vi "Error.Compare Errors with No Error Opt if Same.vi"(7 "No Error if Same":bool=TRUE, 10 "error in2":errorcluster, 11 "error in1":errorcluster) -> (2 "error out":errorcluster, 3 "Same":bool)   [LabVIEW 2018]
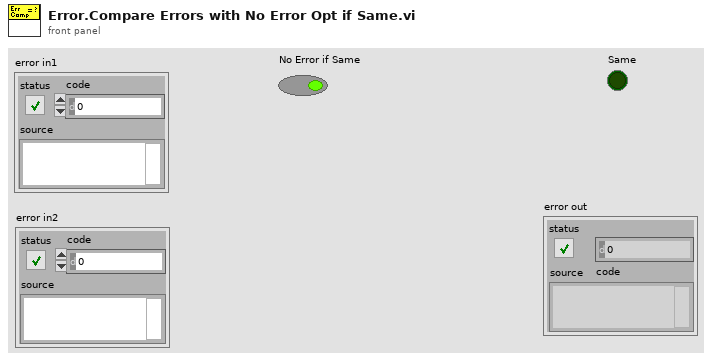
[diagram p1: front panel]
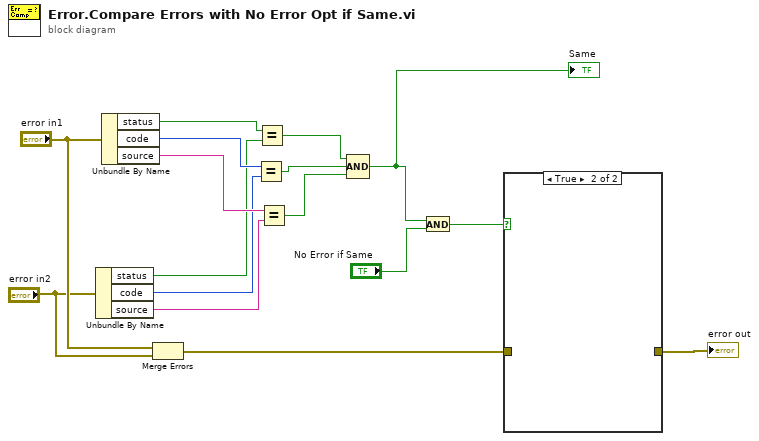
[diagram p0: block diagram]
diagram:
  n1 = Unbundle By Name("error in2") -> ("status"=w13:bool, "code"=w12:i32, "source"=w11:string)
  n2 = Unbundle By Name("error in1") -> ("status"=w16:bool, "code"=w15:i32, "source"=w14:string)
  n3 = Merge Errors("error in1", "error in2") -> (w4:errorcluster)
  n4 = Equal?(x=w15, y=w12) -> (x = y?=w9:bool)
  n5 = Equal?(x=w16, y=w13) -> (x = y?=w10:bool)
  n6 = Equal?(x=w14, y=w11) -> (x = y?=w8:bool)
  n7 = Compound Arithmetic op=AND(w10, w9, w8) -> (w3:bool)
  "Same" <- w3
  n8 = And(x=w3, y="No Error if Same") -> (x .and. y?=w1:bool)
  n9 = case shown="True" w1 {
    tunnel: [w17 _] -> w5
    tunnel: w4 -> [w17 _]
    frame False {
    }
    frame True {
    }
  }
  "error out" <- w5
